vi "Read Container.vi"(8 "error in (no error)":errorcluster, 10 "index":i32, 11 "Storage Line in":refnum<class "Storage Line.lvclass">) -> (0 "error out":errorcluster, 1 "Sample out":refnum<class "Sample.lvclass">, 2 "Containers":T1[](array[typedef]), 3 "Storage Line out":refnum<class "Storage Line.lvclass">)   [LabVIEW 2015, in "cRIO-Carbondioxide.lvlib" / "CO2-Actor.lvlib" / "Storage Line.lvclass"]
uses:
  Storage Line.lvclass
  Controls/Sample Container.ctl
  subs/Sample/Sample.lvclass
  Storage Line.lvclass/Storage Line.ctl
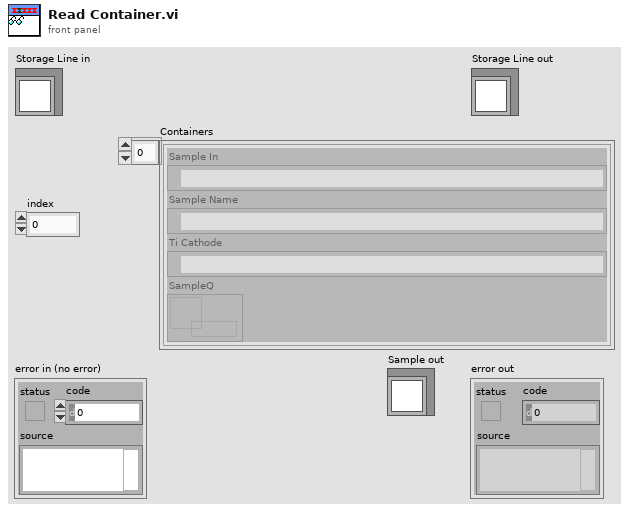
[diagram p1: front panel]
types:
  T1 = typedef "Sample Container.ctl" = cluster{"Sample In":refnum<k21>, "Sample Name":refnum<k21>, "Ti Cathode":refnum<k21>, "SampleQ":refnum<queue>}
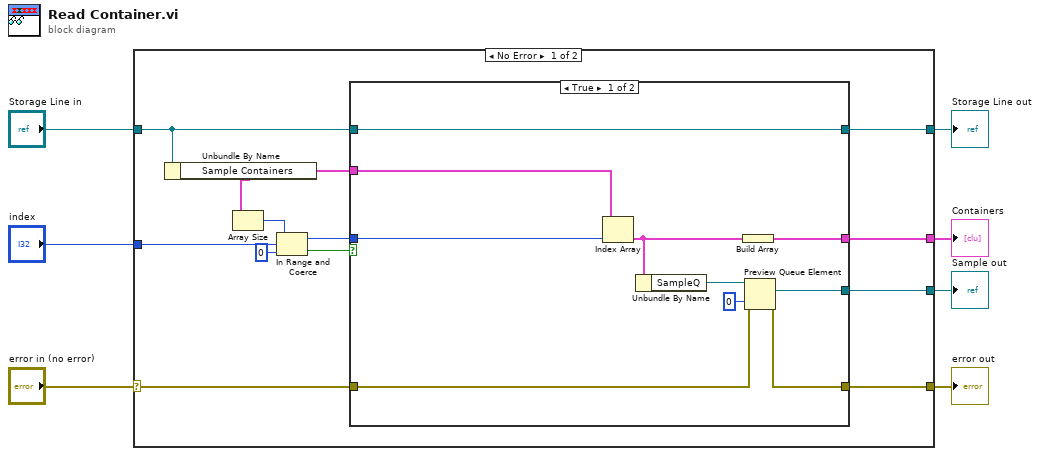
[diagram p0: block diagram]
diagram:
  n1 = case shown="No Error" "error in (no error)" {
    selector: "error in (no error)" -> [w18 w32]
    tunnel: [w17 w32] -> w6
    tunnel: [w15 w33] -> w4
    tunnel: "Storage Line in" -> [w14 w33]
    tunnel: [w16 _] -> w3
    tunnel: "index" -> [w12 _]
    tunnel: [w19 _] -> w1
    frame No Error {
      n2 = Unbundle By Name(w14) -> ("Sample Containers"=w13:T1[])
      n3 = Array Size(array=w13) -> (size(s)=w10:i32)
      n4 = In Range and Coerce(upper limit=w10, x=w12, lower limit=0) -> (coerced(x)=w8:i32, In Range?=w9:bool)
      n5 = case shown="True" w9 {
        tunnel: w14 -> [w22 w31]
        tunnel: [w26 _] -> w19
        tunnel: w18 -> [w25 w30]
        tunnel: [w24 w30] -> w17
        tunnel: [w23 _] -> w16
        tunnel: [w22 w31] -> w15
        tunnel: w13 -> [w21 _]
        tunnel: w8 -> [w20 _]
        frame True {
          n6 = Index Array(array=w21, index=w20) -> (element=w29:T1)
          n7 = Unbundle By Name(w29) -> ("SampleQ"=w27:refnum<queue>)
          n8 = Build Array(w29) -> (w23:T1[])
          n9 = Preview Queue Element(queue=w27, timeout in ms (-1)=0, error in (no error)=w25) -> (element=w26:refnum<class "Sample.lvclass">, error out=w24:errorcluster)  [unwired: 2 out]
        }
        frame False {
        }
      }
    }
    frame Error {
    }
  }
  "error out" <- w6
  "Storage Line out" <- w4
  "Containers" <- w3
  "Sample out" <- w1
